vi "Scratch Parsing VI.vi"() -> ()   [LabVIEW 2014]
uses:
  <vilib>/regexp/Match Regular Expression.xnode
panel:
  out "Numeric":i32
  out "error out":errorcluster
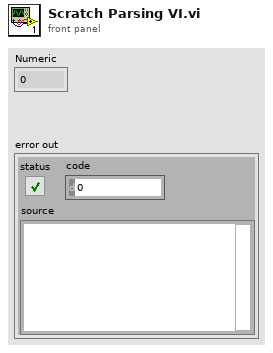
[diagram p1: front panel]
types:
  T1 = enum16{"open", "replace", "create", "open or create", "replace or create", "replace or create with confirmation"}
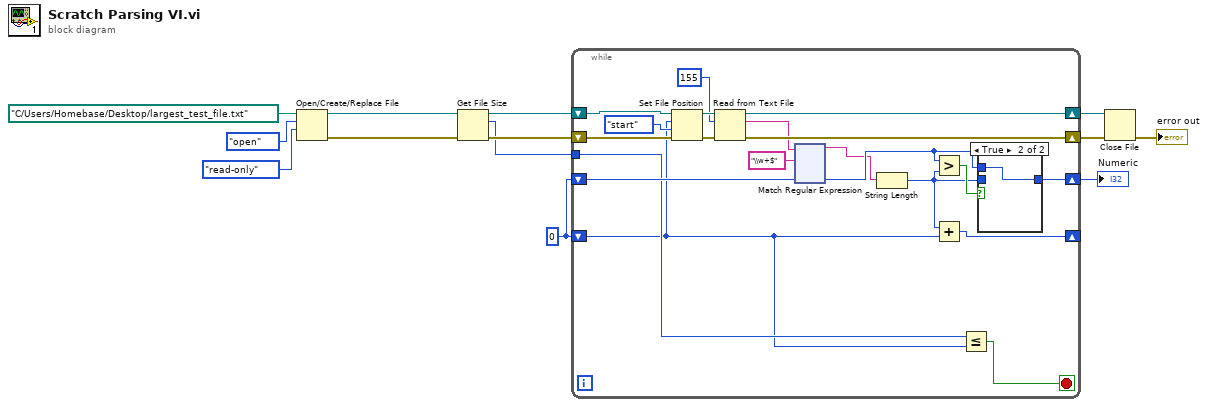
[diagram p0: block diagram]
diagram:
  w7 = 0
  n1 = Open/Create/Replace File(file path (use dialog)=path "C:/Users/Homebase/Desktop/largest_test_file.txt", operation (0:open)=T1."open", access (0:read/write)=enum16{"read/write", "read-only", "write-only"}."read-only") -> (refnum out=w5:refnum<file>, error out=w4:errorcluster)  [unwired: 3 in, 1 out]
  n2 = Get File Size(file=w5, error in=w4) -> (refnum out=w3:refnum<file>, size (in bytes)=w1:i64, 0:w2:errorcluster)
  n3 = while {
    shift-right: [w27] -> w8
    shift-left: w2 -> [w32]
    shift-right: [w28] -> w9
    shift-left: w3 -> [w29]
    shift-right: [w26] -> _
    shift-left: w7 -> [w15]
    shift-right: [w21] -> w6
    shift-left: w7 -> [w20]
    tunnel: w1 -> [w16]
    stop <- w14 stop-if-true
    n4 = Set File Position(offset (in bytes) (0)=w15, refnum=w29, from (0:start)=enum16{"start", "end", "current"}."start", error in=w32) -> (refnum out=w30:refnum<file>, error out=w31:errorcluster)
    n5 = Read from Text File(file (use dialog)=w30, count=155, error in=w31) -> (refnum out=w28:refnum<file>, text=w18:string, error out=w27:errorcluster)  [unwired: 1 in, 1 out]
    n6 = xnode "Match Regular Expression"("input string"=w18, "regular expression"="\\w+$") -> ("before match"=w17:string)  [unwired: 4 in, 4 out]
    n7 = String Length(string=w17) -> (length=w22:i32)
    n8 = Greater?(x=w20, y=w22) -> (0:w23:bool)
    n9 = Add(x=w22, y=w15) -> (x+y=w26:i32)
    n10 = Less Or Equal?(x=w16, y=w15) -> (x <= y?=w14:bool)
    n11 = case shown="True" w23 {
      tunnel: w22 -> [w147 _]
      tunnel: [w147 w148] -> w21
      tunnel: w20 -> [_ w148]
      frame False {
      }
      frame True {
      }
    }
  }
  "Numeric" <- w6
  n12 = Close File(refnum=w9, error in=w8) -> (error out=→"error out":errorcluster)  [unwired: 1 out]
